vi "Get Number Text (inlined).vi"(8 "error in (no error)":errorcluster, 10 "Offset":i32, 11 "JSON":string) -> (0 "error out":errorcluster, 1 "Offset past match":i32, 2 "Number Text":string)   [LabVIEW 2013, in "JSONtext.lvlib"]
uses:
  JSONtext.lvlib
  support/JSONtext support.lvlib
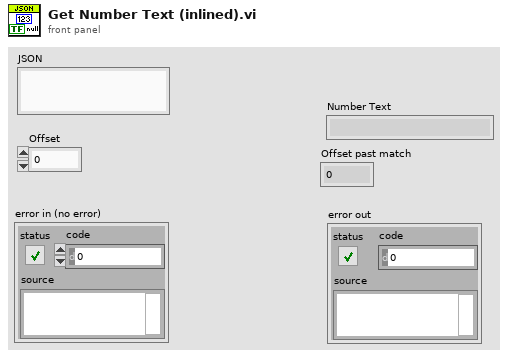
[diagram p1: front panel]
types:
  T1 = typedef "JSONtext.lvlib/Parsing State.ctl" = enum16{"Parser Error", "Object", "Array", "String", "Number/Other", "Leading Whitespace", "Object end", "Array end", "Value end"}
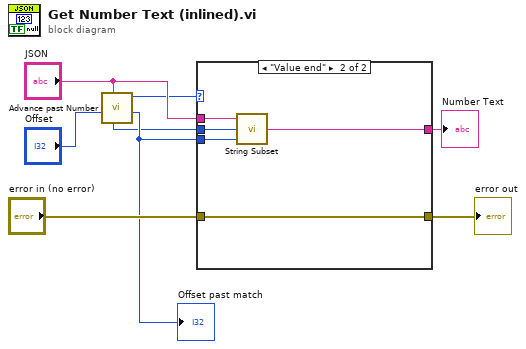
[diagram p0: block diagram]
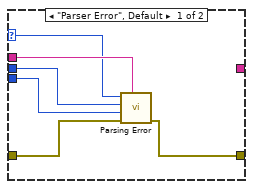
[diagram p2: hidden frame]
diagram:
  n1 = call "Advance past Number.vi"("JSON"="JSON", "Offset (0)"="Offset") -> ("Offset past match"=w3:i32, "Parser State"=w2:T1, "Value start out"=w1:i32)  [unwired: 7 in]
  "Offset past match" <- w3
  n2 = case shown="\"Value end\"" w2 {
    selector: w2 -> [w11 _]
    tunnel: "JSON" -> [w12 w19]
    tunnel: [w14 w15] -> w6
    tunnel: "error in (no error)" -> [w13 w15]
    tunnel: [_ w16] -> w4
    tunnel: w1 -> [w10 w18]
    tunnel: w3 -> [w9 w17]
    frame "Parser Error", Default {
      n3 = call "Parsing Error.vi"("JSON"=w12, "error in (no error)"=w13, "Offset past match"=w9, "Value start"=w10, "State"=w11) -> ("error out"=w14:errorcluster)  [unwired: 6 in]
    }
    frame "Value end" {
      n4 = call "String Subset.vi"("Offset past End"=w17, "Start offset"=w18, "JSON"=w19) -> ("substring"=w16:string)  [unwired: 2 in]
    }
  }
  "error out" <- w6
  "Number Text" <- w4
